vi "Follower16.vi"() -> ()   [LabVIEW 2016]
uses:
  <vilib>/NXT/Block Support/NXT_InputPort.ctl
  <vilib>/NXT/Block Support/NXT_TimerIndex.ctl
  <vilib>/NXT/Block Support/NXT_OutputPort.ctl
  <vilib>/NXT/Dual Mode Library/Sensors/EV3_Gyro_Reset.vi
  <vilib>/NXT/Dual Mode Library/Sensors/EV3_Gyro_Angle.vi
  <vilib>/NXT/Dual Mode Library/Sensors/EV3_Gyro_Rate.vi
  <vilib>/NXT/Dual Mode Library/Sensors/Reset_Timer.vi
  <vilib>/NXT/Dual Mode Library/Sensors/EV3_Color_Reflect.vi
  <vilib>/NXT/Dual Mode Library/Sensors/Read_Timer.vi
  <vilib>/NXT/Dual Mode Library/Sensors/EV3_Ultrasonic_CM.vi
  <vilib>/NXT/Dual Mode Library/Display/drawText_Right.vi
  <vilib>/NXT/Dual Mode Library/prims/inRangeAndCoerce/inRangeAndCoerce_float.vi
  <vilib>/NXT/NXTIO Xnodes/NXTIONodeSubVIs/NXTMoveMotors.vi
  <vilib>/NXT/Dual Mode Library/Display/drawNumber.vi
  <vilib>/NXT/Dual Mode Library/Display/drawNumber_float.vi
  <vilib>/NXT/Dual Mode Library/Motors/Rotation.vi
  <vilib>/NXT/Dual Mode Library/Motors/ResetMotor.vi
  <vilib>/NXT/Dual Mode Library/Sensors/Touch_Pressed.vi
  <vilib>/NXT/Dual Mode Library/Sound/PlayC.vi
  <vilib>/NXT/Dual Mode Library/Display/drawText.vi
  <vilib>/NXT/NXTIO Xnodes/NXTIONodeSubVIs/NXTStopMotors.vi
  <vilib>/NXT/Subs/LVHSConnector.ctl
  <vilib>/NXT/NXTIO Xnodes/AddressXNode/NXTIOAddress.xnode
  <vilib>/NXT/NXTIO Xnodes/NXTIOXNode/NXTIO.xnode
  <vilib>/NXT/LegoClasses/BrickReference/BrickReference.lvclass
panel:
  out "Value (msec)":u32
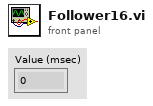
[diagram p1: front panel]
types:
  T1 = typedef "NXT_InputPort.ctl" = u32
  T2 = typedef "LVHSConnector.ctl" = refnum<class "BrickReference.lvclass">
  T3 = typedef "NXT_TimerIndex.ctl" = u8
  T4 = typedef "NXT_OutputPort.ctl" = u8
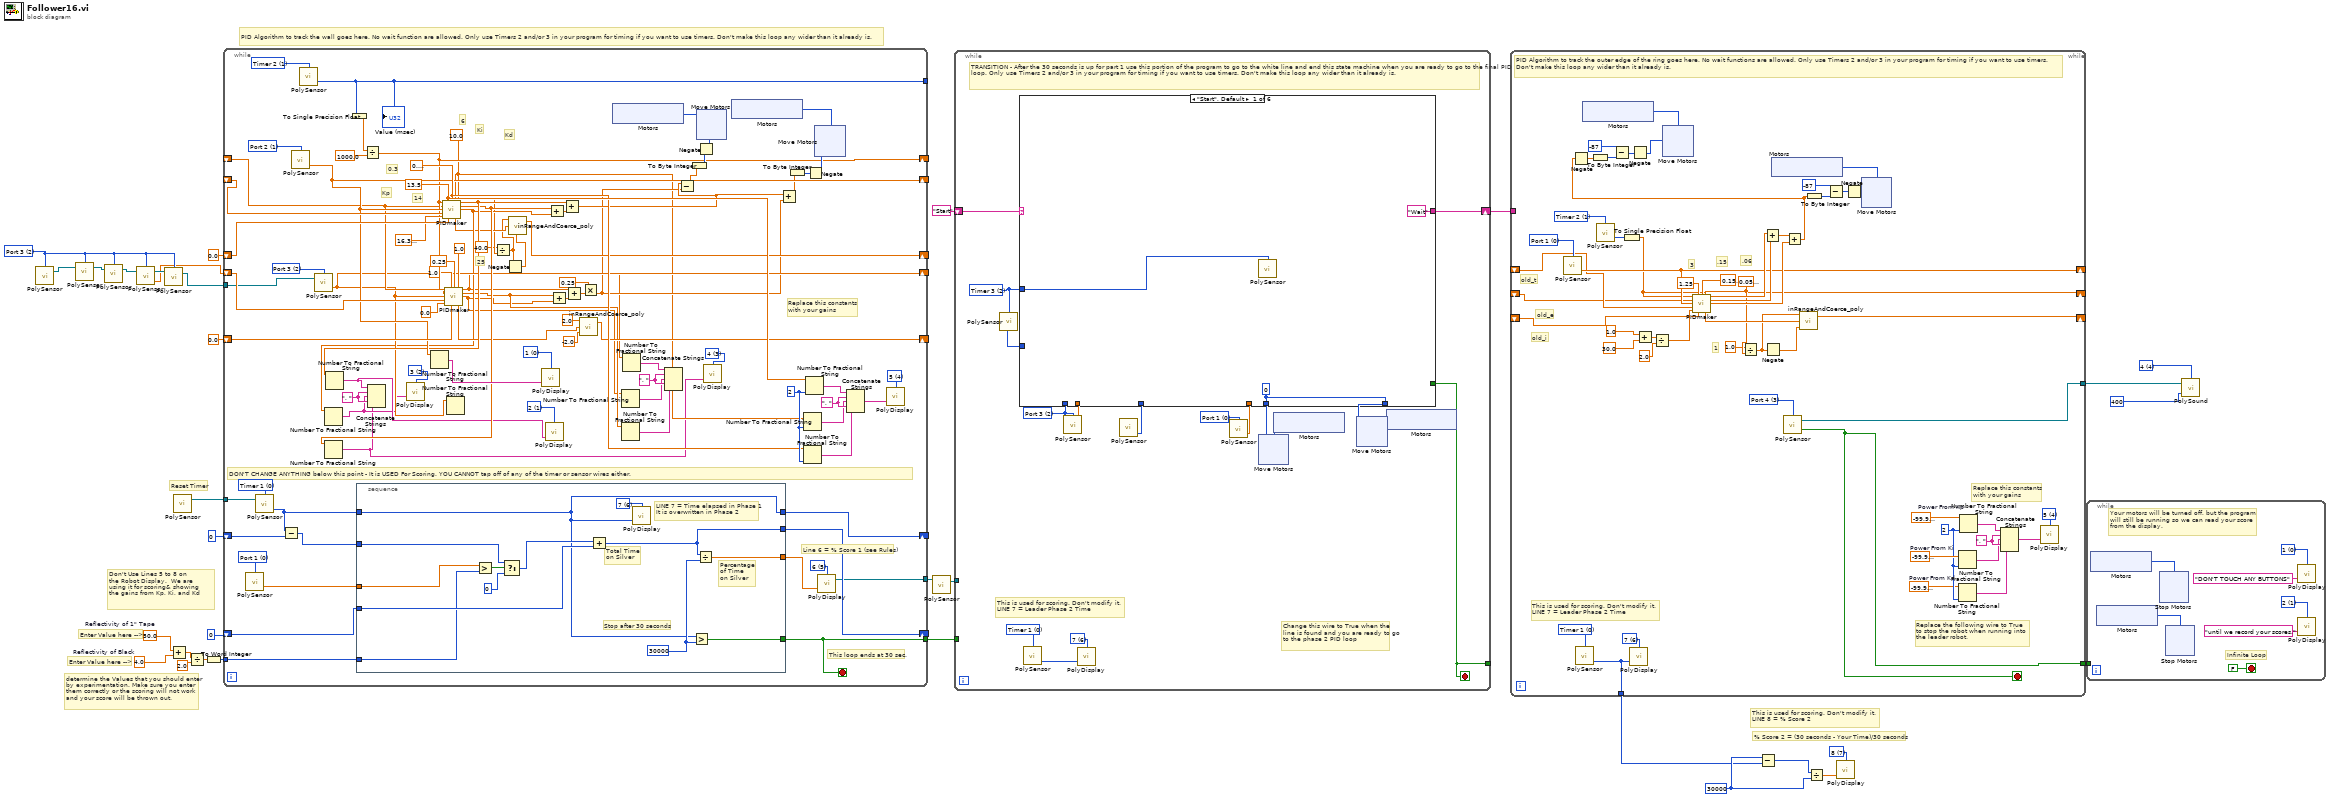
[diagram p0: block diagram]
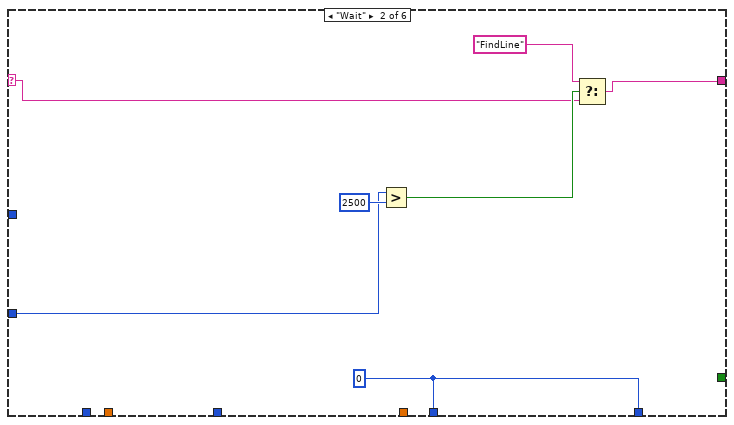
[diagram p2: hidden frame]
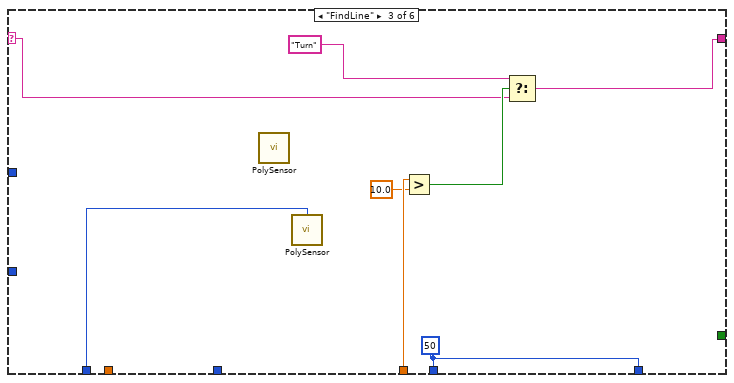
[diagram p3: hidden frame]
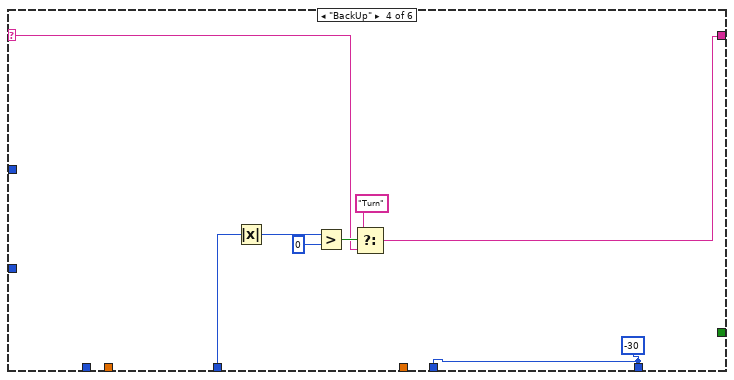
[diagram p4: hidden frame]
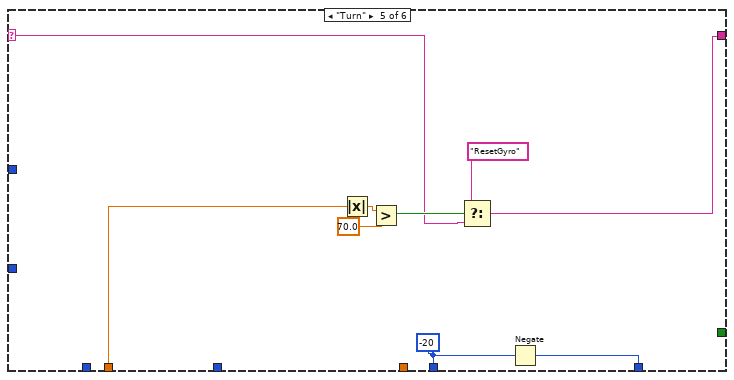
[diagram p5: hidden frame]
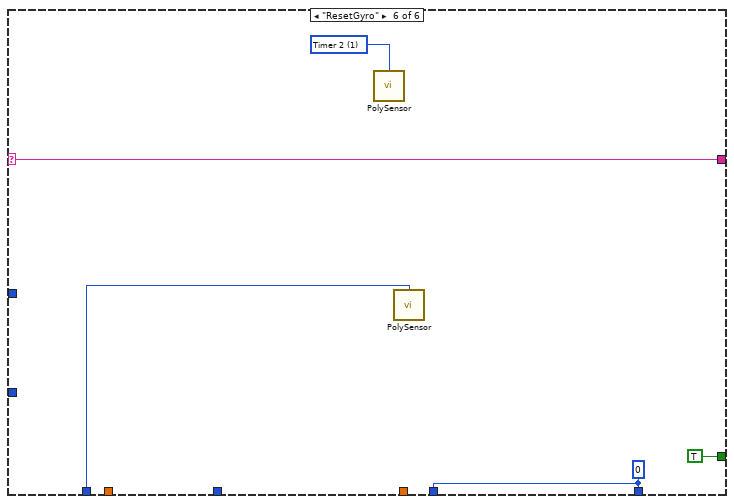
[diagram p6: hidden frame]
diagram:
  w3 = u16 4 items=["3"=3, "4"=4, "5"=5, "6"=6, "7"=7] ("Octave")
  w8 = T1 2 items=["Port 1", "Port 2", "Port 3", "Port 4"] ("Port (Port 1)")
  w16 = u32 30000 ("Value (msec)")
  w17 = i16 7 items=["1", "2", "3", "4", "5", "6", "7", "8", "9", "10", "11", "12"] ("Line")
  w23 = 4.0  # Reflectivity of Black
  w22 = 50.0  # Reflectivity of 1" Tape
  # "PID Algorithm to track the wall goes here. No wait function are allowed. Only use Timers 2 and/or 3 in your program for timing if you want to use timers. Don't make this loop any wider than it already is."
  # "This is used for scoring. Don't modify it.\nLINE 8 = % Score 2"
  # "Don't Use Lines 5 to 8 on\nthe Robot Display.  We are \nusing it for scoring& showing \nthe gains from Kp, Ki, and Kd"
  # "% Score 2 = (30 seconds - Your Time)/30 seconds"
  # "Enter Value here -->"
  # "determine the Values that you should enter\nby experimentation. Make sure you enter \nthem correctly or the scoring will not work\nand your score will be thrown out."
  # "Enter Value here -->"
  # "Reset Timer"
  n1 = call-poly <vilib>:"PolySensor.vi"("Port (Port 1)"=w8) -> ("NXT/EV3"=w9:T2)  [unwired: 3 in]
  n2 = call-poly <vilib>:"PolySensor.vi"("NXT/EV3"=w9, "Port (Port 1)"=w8) -> ("NXT/EV3"=w10:T2)  [unwired: 1 in, 1 out]
  n3 = call-poly <vilib>:"PolySensor.vi"("NXT/EV3"=w10, "Port (Port 1)"=w8) -> ("NXT/EV3"=w12:T2)  [unwired: 1 in, 1 out]
  n4 = call-poly <vilib>:"PolySensor.vi"("NXT/EV3"=w12, "Port (Port 1)"=w8) -> ("Degrees"=w4:sgl, "NXT/EV3"=w11:T2)  [unwired: 1 in]
  n5 = call-poly <vilib>:"PolySensor.vi"("NXT/EV3"=w11, "Port (Port 1)"=w8) -> ("NXT/EV3"=w7:T2)  [unwired: 2 in]
  n6 = Add(x=w22, y=w23) -> (x+y=w21:dbl)
  n7 = call-poly <vilib>:"PolySensor.vi"() -> ("NXT/EV3"=w30:T2)  [unwired: 4 in]
  n8 = Divide(x=w21, y=2.0) -> (x/y=w20:dbl)
  n9 = To Word Integer(number=w20) -> (16bit integer=w27:i16)
  n10 = while {
    shift-right: [w115] -> _
    shift-left: i16 0 -> [w119]
    shift-right: [w116] -> _
    shift-left: i16 0 ("Value (msec)") -> [w118]
    tunnel: w30 -> [w114]
    tunnel: [w117] -> w29
    tunnel: w27 -> [w109]
    tunnel: [w105] -> w25
    shift-right: [w50] -> _
    shift-left: sgl 0.0 ("coerced(x)") -> [w86]
    shift-right: [w65] -> _
    shift-left: sgl 0.0 ("coerced(x)") -> [w91]
    shift-right: [w54] -> _
    shift-left: w4 -> [w89]
    tunnel: [w85] -> _
    shift-right: [w60] -> _
    shift-left: _ -> [w59]
    shift-right: [w73] -> _
    shift-left: _ -> [w81]
    tunnel: w7 -> [w53]
    stop <- w117 stop-if-true
    w46 = ", " ("string")
    w43 = i16 3 items=["1", "2", "3", "4", "5", "6", "7", "8", "9", "10", "11", "12"] ("Line")
    w55 = i16 1 items=["1", "2", "3", "4", "5", "6", "7", "8", "9", "10", "11", "12"] ("Line")
    w72 = ", " ("string")
    w71 = i16 2 items=["1", "2", "3", "4", "5", "6", "7", "8", "9", "10", "11", "12"] ("Line")
    w75 = i16 0 items=["1", "2", "3", "4", "5", "6", "7", "8", "9", "10", "11", "12"] ("Line")
    w39 = sgl 10.0 ("Ki")
    w78 = sgl 0.3 ("Kd")
    w79 = sgl 13.5 ("Kp")
    w82 = T1 1 items=["Port 1", "Port 2", "Port 3", "Port 4"] ("Port (Port 1)")
    w87 = T3 1 items=["Timer 1", "Timer 2", "Timer 3"] ("Timer (Timer 1)")
    w90 = T1 2 items=["Port 1", "Port 2", "Port 3", "Port 4"] ("Port (Port 1)")
    w101 = ", " ("string")
    w103 = i16 2 ("precision (6)")
    w104 = i16 4 items=["1", "2", "3", "4", "5", "6", "7", "8", "9", "10", "11", "12"] ("Line")
    w107 = i16 5 items=["1", "2", "3", "4", "5", "6", "7", "8", "9", "10", "11", "12"] ("Line")
    w111 = T1 0 items=["Port 1", "Port 2", "Port 3", "Port 4"] ("Port (Port 3)")
    w112 = T3 0 items=["Timer 1", "Timer 2", "Timer 3"] ("Timer (Timer 1)")
    # "14"
    # "25"
    # "6"
    # "0.3"
    # "Kp"
    # "Kd"
    # "Ki"
    # "Replace this constants\nwith your gains"
    # "DON'T CHANGE ANYTHING below this point - It is USED For Scoring. YOU CANNOT tap off of any of the timer or sensor wires either."
    # "Line 6 = % Score 1 (see Rules)"
    # "This loop ends at 30 sec."
    n11 = call-poly <vilib>:"PolySensor.vi"("Port (Port 1)"=w111) -> ("Scaled Value"=w110:sgl)  [unwired: 2 in, 1 out]
    n12 = call-poly <vilib>:"PolySensor.vi"("NXT/EV3"=w114, "Timer (Timer 1)"=w112) -> ("Value (msec)"=w113:u32)  [unwired: 1 in, 1 out]
    n13 = Subtract(x=w113, y=w118) -> (x-y=w108:u32)
    n14 = call-poly <vilib>:"PolySensor.vi"("Port (Port 1)"=w82) -> ("Centimeters"=w73:sgl)  [unwired: 2 in, 1 out]
    n15 = call-poly <vilib>:"PolySensor.vi"("Timer (Timer 1)"=w87) -> ("Value (msec)"=w85:u32)  [unwired: 2 in, 1 out]
    "Value (msec)" <- w85
    n16 = call-poly <vilib>:"PolySensor.vi"("NXT/EV3"=w53, "Port (Port 1)"=w90) -> ("Degrees"=w54:sgl)  [unwired: 1 in, 1 out]
    n17 = To Single Precision Float(number=w85) -> (single precision float=w83:sgl)
    n18 = stacked-sequence {
      tunnel: w119 -> [w148]
      tunnel: [w138] -> w106
      tunnel: w113 -> [w136]
      tunnel: [w147] -> w117
      tunnel: w110 -> [w142]
      tunnel: w108 -> [w144]
      tunnel: [w136] -> w116
      tunnel: [w140] -> w115
      tunnel: w109 -> [w141]
      frame #0 {
        w137 = i16 6 items=["1", "2", "3", "4", "5", "6", "7", "8", "9", "10", "11", "12"] ("Line")
        w139 = u32 30000 ("Value (msec)")
        # "LINE 7 = Time elapsed in Phase 1\nIt is overwritten in Phase 2"
        # "Percentage\nof Time\non Silver"
        # "Stop after 30 seconds"
        # "Total Time\non Silver"
        n19 = Greater?(x=w142, y=w141) -> (0:w145:bool)
        n20 = Select(t=w144, s=w145, f=i16 0) -> (s? t:f=w143:u32)
        n21 = Add(x=w143, y=w148) -> (x+y=w140:u32)
        n22 = call-poly <vilib>:"PolyDisplay.vi"("number"=w136, "Line"=w137) -> ()  [unwired: 2 in, 1 out]
        n23 = Greater?(x=w136, y=w139) -> (0:w147:bool)
        n24 = Divide(x=w140, y=w139) -> (x/y=w138:dbl)
      }
    }
    n25 = Divide(x=w83, y=sgl 1000.0) -> (x/y=w60:sgl)
    n26 = Number To Fractional String(number=w73) -> (F-format string=w74:string)  [unwired: 3 in]
    n27 = call "PIDmaker.vi"("New Time"=w60, "Kp"=w79, "Kd"=w78, "Ki"=w39, "Old Time"=w59, "New Value"=w73, "Old Value"=w81, "Desired Value"=sgl 16.4, "Integral In"=w86) -> ("P out"=w70:sgl, "D out"=w69:sgl, "I out"=w52:sgl, "Integral Out"=w51:sgl)  [unwired: 3 in]
    n28 = Number To Fractional String(number=w52) -> (F-format string=w34:string)  [unwired: 3 in]
    n29 = Number To Fractional String(number=w69) -> (F-format string=w33:string)  [unwired: 3 in]
    n30 = Number To Fractional String(number=w70) -> (F-format string=w35:string)  [unwired: 3 in]
    n31 = Concatenate Strings(w35, w72, w34, w72, w33) -> ()  [unwired: 1 out]
    n32 = call-poly <vilib>:"PolyDisplay.vi"("Text"=w34, "Line"=w71) -> ()  [unwired: 2 in, 1 out]
    n33 = call "PIDmaker.vi"("New Time"=w60, "Kp"=sgl 1.0, "Kd"=sgl 0.25, "Ki"=sgl 1.0, "Old Time"=w59, "New Value"=w54, "Old Value"=w89, "Desired Value"=sgl 0.0, "Integral In"=w91) -> ("P out"=w42:sgl, "D out"=w41:sgl, "I out"=w40:sgl, "Integral Out"=w66:sgl)  [unwired: 3 in]
    n34 = Number To Fractional String(number=w54) -> ()  [unwired: 3 in, 1 out]
    n35 = Divide(x=sgl 40.0, y=w39) -> (x/y=w37:sgl)
    n36 = Negate(x=w37) -> (-x=w36:sgl)
    n37 = call-poly <vilib>:"inRangeAndCoerce_poly.vi"("lower limit"=w36, "x"=w51, "upper limit"=w37) -> ("coerced(x)"=w50:sgl)  [unwired: 1 out]
    n38 = call-poly <vilib>:"PolyDisplay.vi"("Text"=w74, "Line"=w75) -> ()  [unwired: 2 in, 1 out]
    n39 = call-poly <vilib>:"PolyDisplay.vi"("Text"=w35, "Line"=w55) -> ()  [unwired: 2 in, 1 out]
    n40 = Add(x=w69, y=w52) -> (x+y=w95:sgl)
    n41 = Add(x=w41, y=w40) -> (x+y=w92:sgl)
    n42 = Add(x=w70, y=w95) -> (x+y=w63:sgl)
    n43 = Add(x=w42, y=w92) -> (x+y=w61:sgl)
    n44 = call-poly <vilib>:"inRangeAndCoerce_poly.vi"("lower limit"=sgl -2.0, "x"=w66, "upper limit"=sgl 2.0) -> ("coerced(x)"=w65:sgl)  [unwired: 1 out]
    n45 = Multiply(x=sgl 0.25, y=w61) -> (x*y=w49:sgl)
    n46 = xnode "Motors"() -> ("Motor"=w97:T4)
    n47 = Number To Fractional String(number=w40) -> (F-format string=w45:string)  [unwired: 3 in]
    n48 = Number To Fractional String(number=w41) -> (F-format string=w44:string)  [unwired: 3 in]
    n49 = Number To Fractional String(number=w42) -> (F-format string=w47:string)  [unwired: 3 in]
    n50 = Concatenate Strings(w47, w46, w45, w46, w44) -> ()  [unwired: 1 out]
    n51 = Subtract(x=w63, y=w49) -> (x-y=w64:sgl)
    n52 = To Byte Integer(number=w64) -> (8bit integer=w76:i8)
    n53 = Negate(x=w76) -> (-x=w68:i8)
    n54 = xnode "Move Motors"("Power/Speed 1"=w68, "Motors"=w97) -> ()  [unwired: 1 in, 1 out]
    n55 = call-poly <vilib>:"PolyDisplay.vi"("Text"=w33, "Line"=w43) -> ()  [unwired: 2 in, 1 out]
    n56 = xnode "Motors"() -> ("Motor"=w96:T4)
    n57 = Add(x=w63, y=w49) -> (x+y=w62:sgl)
    n58 = To Byte Integer(number=w62) -> (8bit integer=w77:i8)
    n59 = Number To Fractional String(number=w39, precision (6)=w103) -> (F-format string=w100:string)  [unwired: 2 in]
    n60 = Number To Fractional String(number=w78, precision (6)=w103) -> (F-format string=w99:string)  [unwired: 2 in]
    n61 = Number To Fractional String(number=w79, precision (6)=w103) -> (F-format string=w102:string)  [unwired: 2 in]
    n62 = Negate(x=w77) -> (-x=w67:i8)
    n63 = xnode "Move Motors"("Power/Speed 1"=w67, "Motors"=w96) -> ()  [unwired: 1 in, 1 out]
    n64 = call-poly <vilib>:"PolyDisplay.vi"("number"=w106, "Line"=w107) -> ("NXT/EV3"=w105:T2)  [unwired: 2 in]
    n65 = Concatenate Strings(w102, w101, w100, w101, w99) -> (w98:string)
    n66 = call-poly <vilib>:"PolyDisplay.vi"("Text"=w98, "Line"=w104) -> ()  [unwired: 2 in, 1 out]
  }
  n67 = call-poly <vilib>:"PolySensor.vi"("NXT/EV3"=w25) -> ("NXT/EV3"=w24:T2)  [unwired: 3 in]
  n68 = while {
    tunnel: w29 -> [_]
    shift-right: [w151] -> w18
    shift-left: "Start" -> [w150]
    tunnel: w24 -> [_]
    tunnel: [w149] -> _
    stop <- w149 stop-if-true
    w154 = T1 2 items=["Port 1", "Port 2", "Port 3", "Port 4"] ("Port (Port 1)")
    w156 = T1 0 items=["Port 1", "Port 2", "Port 3", "Port 4"] ("Port (Port 1)")
    w160 = T3 2 items=["Timer 1", "Timer 2", "Timer 3"] ("Timer (Timer 1)")
    w163 = i16 6 items=["1", "2", "3", "4", "5", "6", "7", "8", "9", "10", "11", "12"] ("Line")
    w165 = T3 0 items=["Timer 1", "Timer 2", "Timer 3"] ("Timer (Timer 1)")
    # "This is used for scoring. Don't modify it.\nLINE 7 = Leader Phase 2 Time"
    # "Change this wire to True when the line is found and you are ready to go to the phase 2 PID loop"
    # "TRANSITION - After the 30 seconds is up for part 1 use this portion of the program to go to the white line and end this state machine when you are ready to go to the final PID control loop. Only use Timers 2 and/or 3 in your program for timing if you want to use timers. Don't make this loop any wider than it already is."
    n69 = call-poly <vilib>:"PolySensor.vi"("Timer (Timer 1)"=w160) -> ("Value (msec)"=w159:u32)  [unwired: 2 in, 1 out]
    n70 = call-poly <vilib>:"PolySensor.vi"("Timer (Timer 1)"=w165) -> ("Value (msec)"=w164:u32)  [unwired: 2 in, 1 out]
    n71 = call-poly <vilib>:"PolySensor.vi"("Port (Port 1)"=w154) -> ("Degrees"=w153:sgl)  [unwired: 2 in, 1 out]
    n72 = call-poly <vilib>:"PolyDisplay.vi"("number"=w164, "Line"=w163) -> ()  [unwired: 2 in, 1 out]
    n73 = call-poly <vilib>:"PolySensor.vi"() -> ("Angle of Rotation"=w152:i32)  [unwired: 3 in, 1 out]
    n74 = call-poly <vilib>:"PolySensor.vi"("Port (Port 1)"=w156) -> ("Scaled Value"=w155:sgl)  [unwired: 2 in, 1 out]
    n75 = case shown="\"Start\", Default" w150 {
      selector: w150 -> [_ w187 w194 w202 w209 w219]
      tunnel: ["Wait" w190 w196 w200 w208 w219] -> w151
      tunnel: w160 -> [w184 _ _ _ _ _]
      tunnel: w159 -> [_ w186 _ _ _ _]
      tunnel: [w182 w185 w192 w207 w216 w218] -> w158
      tunnel: [w182 w185 w192 w207 w215 w218] -> w157
      tunnel: w155 -> [_ _ w199 _ _ _]
      tunnel: w154 -> [_ _ w193 _ _ w221]
      tunnel: w153 -> [_ _ _ _ w214 _]
      tunnel: w152 -> [_ _ _ w206 _ _]
      tunnel: [_ _ _ _ _ TRUE] -> w149
      frame "Start", Default {
        w182 = 0
        n76 = call-poly <vilib>:"PolySensor.vi"("Timer (Timer 1)"=w184) -> ()  [unwired: 3 in, 1 out]
      }
      frame "Wait" {
        w185 = 0
        n77 = Greater?(x=w186, y=u32 2500) -> (0:w188:bool)
        n78 = Select(t="FindLine", s=w188, f=w187) -> (s? t:f=w190:string)
      }
      frame "FindLine" {
        w192 = 50
        n79 = call-poly <vilib>:"PolySensor.vi"() -> ()  [unwired: 4 in, 1 out]
        n80 = call-poly <vilib>:"PolySensor.vi"("Port (Port 1)"=w193) -> ()  [unwired: 3 in, 1 out]
        n81 = Greater?(x=w199, y=sgl 10.0) -> (0:w197:bool)
        n82 = Select(t="Turn", s=w197, f=w194) -> (s? t:f=w196:string)
      }
      frame "BackUp" {
        w207 = -30
        n83 = Absolute Value(x=w206) -> (abs(x)=w204:i32)
        n84 = Greater?(x=w204, y=0) -> (0:w203:bool)
        n85 = Select(t="Turn", s=w203, f=w202) -> (s? t:f=w200:string)
      }
      frame "Turn" {
        w216 = -20
        n86 = Absolute Value(x=w214) -> (abs(x)=w213:sgl)
        n87 = Greater?(x=w213, y=sgl 70.0) -> (0:w211:bool)
        n88 = Select(t="ResetGyro", s=w211, f=w209) -> (s? t:f=w208:string)
        n89 = Negate(x=w216) -> (-x=w215:i32)
      }
      frame "ResetGyro" {
        w217 = T3 1 items=["Timer 1", "Timer 2", "Timer 3"] ("Timer (Timer 1)")
        w218 = 0
        n90 = call-poly <vilib>:"PolySensor.vi"("Timer (Timer 1)"=w217) -> ()  [unwired: 3 in, 1 out]
        n91 = call-poly <vilib>:"PolySensor.vi"("Port (Port 1)"=w221) -> ()  [unwired: 3 in, 1 out]
      }
    }
    n92 = xnode "Motors"() -> ("Motor"=w162:T4)
    n93 = xnode "Move Motors"("Power/Speed 1"=w158, "Motors"=w162) -> ()  [unwired: 1 in, 1 out]
    n94 = xnode "Motors"() -> ("Motor"=w161:T4)
    n95 = xnode "Move Motors"("Power/Speed 1"=w157, "Motors"=w161) -> ()  [unwired: 1 in, 1 out]
  }
  n96 = while {
    tunnel: [w230] -> w19
    tunnel: w18 -> [_]
    tunnel: [w272] -> w15
    shift-right: [w237] -> _
    shift-left: _ -> [w233]
    shift-right: [w236] -> _
    shift-left: _ -> [w232]
    shift-right: [w235] -> _
    shift-left: _ -> [w234]
    tunnel: [w222] -> w1
    stop <- w230 stop-if-true
    w231 = T1 3 items=["Port 1", "Port 2", "Port 3", "Port 4"] ("Port (Port 1)")
    w245 = sgl 0.05 ("Ki")
    w259 = T3 1 items=["Timer 1", "Timer 2", "Timer 3"] ("Timer (Timer 1)")
    w260 = T1 0 items=["Port 1", "Port 2", "Port 3", "Port 4"] ("Port (Port 1)")
    w265 = ", " ("string")
    w268 = i16 2 ("precision (6)")
    w267 = sgl -99.9  # Power From Kd
    w269 = sgl -99.9  # Power From Ki
    w270 = sgl -99.9  # Power From Kp
    w271 = i16 4 items=["1", "2", "3", "4", "5", "6", "7", "8", "9", "10", "11", "12"] ("Line")
    w273 = i16 6 items=["1", "2", "3", "4", "5", "6", "7", "8", "9", "10", "11", "12"] ("Line")
    w274 = T3 0 items=["Timer 1", "Timer 2", "Timer 3"] ("Timer (Timer 1)")
    # "3"
    # ".15"
    # ".06"
    # "1"
    # "old_i"
    # "old_e"
    # "old_t"
    # "Replace this constants\nwith your gains"
    # "This is used for scoring. Don't modify it.\nLINE 7 = Leader Phase 2 Time"
    # "PID Algorithm to track the outer edge of the ring goes here. No wait functions are allowed. Only use Timers 2 and/or 3 in your program for timing if you want to use timers.\nDon't make this loop any wider than it already is."
    # "Replace the following wire to True\nto stop the robot when running into \nthe leader robot."
    n97 = call-poly <vilib>:"PolySensor.vi"("Port (Port 1)"=w260) -> ("Scaled Value"=w237:sgl)  [unwired: 2 in, 1 out]
    n98 = call-poly <vilib>:"PolySensor.vi"("Timer (Timer 1)"=w274) -> ("Value (msec)"=w272:u32)  [unwired: 2 in, 1 out]
    n99 = xnode "Motors"() -> ("Motor"=w242:T4)
    n100 = call-poly <vilib>:"PolySensor.vi"("Timer (Timer 1)"=w259) -> ("Value (msec)"=w258:u32)  [unwired: 2 in, 1 out]
    n101 = To Single Precision Float(number=w258) -> (single precision float=w236:sgl)
    n102 = call-poly <vilib>:"PolyDisplay.vi"("number"=w272, "Line"=w273) -> ()  [unwired: 2 in, 1 out]
    n103 = Add(x=sgl 1.0, y=sgl 30.0) -> (x+y=w255:sgl)
    n104 = Divide(x=w255, y=sgl 2.0) -> (x/y=w252:sgl)
    n105 = call "PIDmaker.vi"("New Time"=w236, "Kp"=sgl 1.25, "Kd"=sgl 0.15, "Ki"=w245, "Old Time"=w232, "New Value"=w237, "Old Value"=w233, "Desired Value"=w252, "Integral In"=w234) -> ("P out"=w248:sgl, "D out"=w247:sgl, "I out"=w246:sgl, "Integral Out"=w251:sgl)  [unwired: 3 in]
    n106 = Divide(x=sgl 1.0, y=w245) -> (x/y=w243:sgl)
    n107 = Add(x=w248, y=w247) -> (x+y=w249:sgl)
    n108 = Negate(x=w243) -> (-x=w244:sgl)
    n109 = xnode "Motors"() -> ("Motor"=w261:T4)
    n110 = call-poly <vilib>:"PolySensor.vi"("Port (Port 1)"=w231) -> ("Yes / No"=w230:bool, "NXT/EV3"=w222:T2)  [unwired: 2 in]
    n111 = Add(x=w249, y=w246) -> (x+y=w224:sgl)
    n112 = Negate(x=w224) -> (-x=w225:sgl)
    n113 = To Byte Integer(number=w225) -> (8bit integer=w229:i8)
    n114 = Subtract(x=i8 -87, y=w229) -> (x-y=w227:i8)
    n115 = Negate(x=w227) -> (-x=w226:i8)
    n116 = xnode "Move Motors"("Power/Speed 1"=w226, "Motors"=w242) -> ()  [unwired: 1 in, 1 out]
    n117 = call-poly <vilib>:"inRangeAndCoerce_poly.vi"("lower limit"=w244, "x"=w251, "upper limit"=w243) -> ("coerced(x)"=w235:sgl)  [unwired: 1 out]
    n118 = To Byte Integer(number=w224) -> (8bit integer=w241:i8)
    n119 = Subtract(x=i8 -87, y=w241) -> (x-y=w239:i8)
    n120 = Negate(x=w239) -> (-x=w238:i8)
    n121 = xnode "Move Motors"("Power/Speed 1"=w238, "Motors"=w261) -> ()  [unwired: 1 in, 1 out]
    n122 = Number To Fractional String(number=w269, precision (6)=w268) -> (F-format string=w264:string)  [unwired: 2 in]
    n123 = Number To Fractional String(number=w267, precision (6)=w268) -> (F-format string=w263:string)  [unwired: 2 in]
    n124 = Number To Fractional String(number=w270, precision (6)=w268) -> (F-format string=w266:string)  [unwired: 2 in]
    n125 = Concatenate Strings(w266, w265, w264, w265, w263) -> (w262:string)
    n126 = call-poly <vilib>:"PolyDisplay.vi"("Text"=w262, "Line"=w271) -> ()  [unwired: 2 in, 1 out]
  }
  n127 = Subtract(x=w16, y=w15) -> (x-y=w14:u32)
  n128 = Divide(x=w14, y=w16) -> (x/y=w13:dbl)
  n129 = call-poly <vilib>:"PolyDisplay.vi"("number"=w13, "Line"=w17) -> ()  [unwired: 2 in, 1 out]
  n130 = while {
    tunnel: w19 -> [_]
    stop <- FALSE stop-if-true
    w291 = i16 1 items=["1", "2", "3", "4", "5", "6", "7", "8", "9", "10", "11", "12"] ("Line")
    w294 = i16 0 items=["1", "2", "3", "4", "5", "6", "7", "8", "9", "10", "11", "12"] ("Line")
    # "Your motors will be turned off, but the program\nwill still be running so we can read your score\nfrom the display."
    # "Infinite Loop"
    n131 = xnode "Motors"() -> ("Motor"=w296:T4)
    n132 = xnode "Motors"() -> ("Motor"=w295:T4)
    n133 = xnode "Stop Motors"("Motors"=w296) -> ()  [unwired: 1 in, 1 out]
    n134 = xnode "Stop Motors"("Motors"=w295) -> ()  [unwired: 1 in, 1 out]
    n135 = call-poly <vilib>:"PolyDisplay.vi"("Text"="DON'T TOUCH ANY BUTTONS", "Line"=w294) -> ()  [unwired: 2 in, 1 out]
    n136 = call-poly <vilib>:"PolyDisplay.vi"("Text"="until we record your scores.", "Line"=w291) -> ()  [unwired: 2 in, 1 out]
  }
  n137 = call-poly <vilib>:"PolySound.vi"("Duration (500 ms)"=u16 400, "NXT/EV3"=w1, "Octave"=w3) -> ()  [unwired: 1 in, 1 out]
